vi "Generate Z-Stack Image references.vi"(8 "error in (no error)":errorcluster, 9 "IMAQ reference name":string, 10 "Channel File Names":string[](array[string]), 11 "Channel File Paths":path[](array[path])) -> (0 "error out":errorcluster, 2 "Image Array refs":T1[](array[typedef]), 3 "MaxZ":T1)   [LabVIEW 2020]
uses:
  <vilib>/vision/Image Controls.llb/IMAQ Image.ctl
  <vilib>/vision/NI_Vision_Development_Module.lvlib
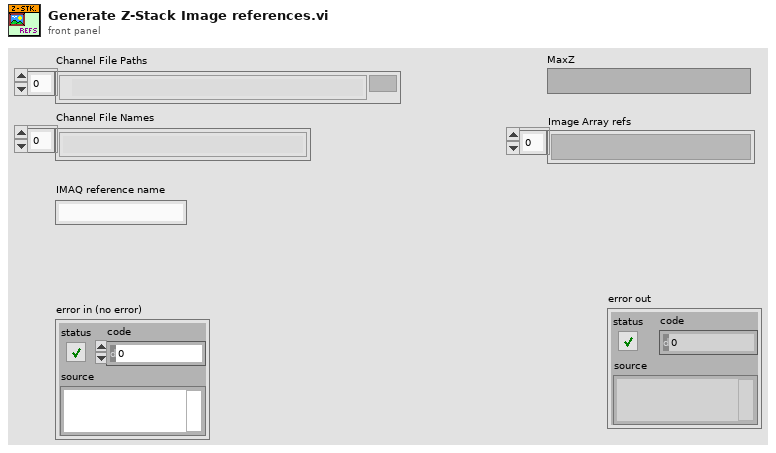
[diagram p1: front panel]
types:
  T1 = typedef "IMAQ Image.ctl" = refnum<image>
  T2 = typedef "Image Type" = u32
  T3 = enum32{"Average", "Min", "Max", "Clear  if < ", "Clear  if < or =", "Clear  if =", "Clear  if > or =", "Clear  if >"}
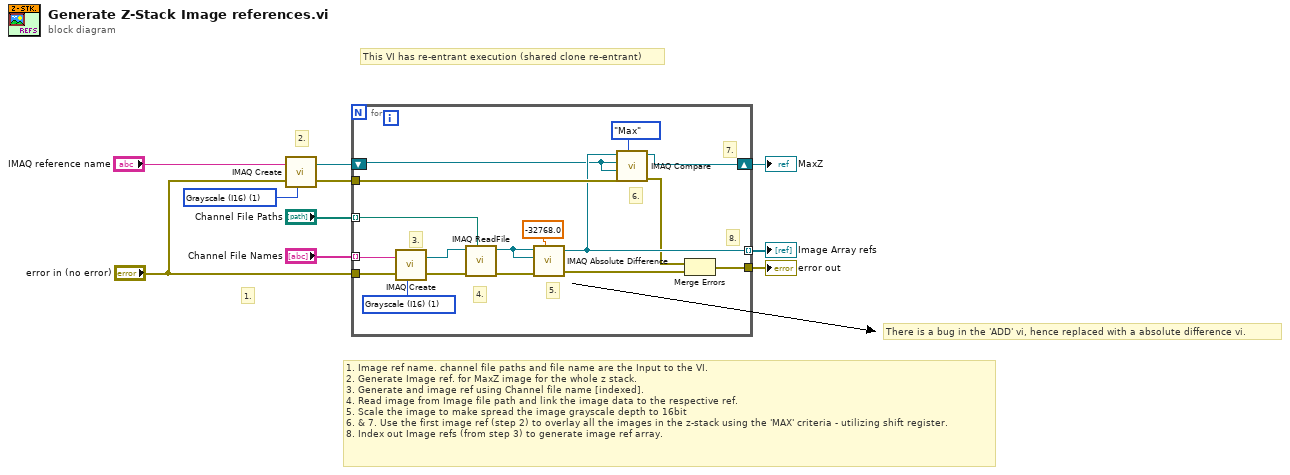
[diagram p0: block diagram]
diagram:
  w1 = T2 1 items=["Grayscale (U8)", "Grayscale (I16)", "Grayscale (SGL)", "Complex (CSG)", "RGB (U32)", "HSL (U32)", "RGB (U64)", "Grayscale (U16)"] ("Image Type")
  # "There is a bug in the 'ADD' vi, hence replaced with a absolute difference vi."
  # "1."
  # "1. Image ref name. channel file paths and file name are the Input to the VI. \n2. Generate Image ref. for MaxZ image for the whole z stack.\n3. Generate and image ref using Channel file name [indexed].\n4. Read image from Image file path and link the image data to the respective ref.\n5. Scale the image to make spread the image grayscale depth to 16bit\n6. & 7. Use the first image ref (step 2) to overlay all the images in the z-stack using the 'MAX' criteria - utilizing shift register.\n8. Index out Image refs (from step 3) to generate image ref array."
  # "2."
  # "This VI has re-entrant execution (shared clone re-entrant)"
  n1 = call "IMAQ Create"("Image Name"="IMAQ reference name", "Image Type"=w1, "error in (no error)"="error in (no error)") -> ("New Image"=w7:T1, "error out"=w5:errorcluster)  [unwired: 2 in]
  n2 = for {
    tunnel: "Channel File Names" -> [w26] mode=indexing
    tunnel: "Channel File Paths" -> [w22] mode=indexing
    shift-right: [w14] -> w3
    shift-left: w7 -> [w15]
    tunnel: "error in (no error)" -> [w25]
    tunnel: [w16] -> w2 mode=indexing
    tunnel: w5 -> [w17]
    tunnel: [w11] -> w4
    w27 = T2 1 items=["Grayscale (U8)", "Grayscale (I16)", "Grayscale (SGL)", "Complex (CSG)", "RGB (U32)", "HSL (U32)", "RGB (U64)"] ("Image Type")
    # "7."
    # "8."
    # "6."
    # "5."
    # "4."
    # "3."
    n3 = call "IMAQ Create"("Image Name"=w26, "Image Type"=w27, "error in (no error)"=w25) -> ("New Image"=w23:T1, "error out"=w24:errorcluster)  [unwired: 2 in]
    n4 = call "IMAQ ReadFile"("File Path"=w22, "error in (no error)"=w24, "Image"=w23) -> ("error out"=w19:errorcluster, "Image Out"=w18:T1)  [unwired: 4 in, 3 out]
    n5 = call "IMAQ Absolute Difference"("Image Src A"=w18, "Constant"=-32768.0, "Image Dst"=w18, "error in (no error)"=w19) -> ("Image Dst Out"=w16:T1, "error out"=w12:errorcluster)  [unwired: 3 in]
    n6 = call "IMAQ Compare"("Operator"=T3."Max", "error in (no error)"=w17, "Image Src B"=w15, "Image Dst"=w15, "Image Src A"=w16) -> ("error out"=w13:errorcluster, "Image Dst Out"=w14:T1)  [unwired: 5 in]
    n7 = Merge Errors(w13, w12) -> (w11:errorcluster)
  }
  "error out" <- w4
  "MaxZ" <- w3
  "Image Array refs" <- w2
